vi "Timer Reset.vi"(8 "error in (no error)":errorcluster, 11 "LV Server in":refnum<class "LV Server.lvclass">) -> (0 "error out":errorcluster, 3 "LV Server out":refnum<class "LV Server.lvclass">)   [LabVIEW 2020, in "LV Server.lvclass"]
uses:
  LV Server.lvclass
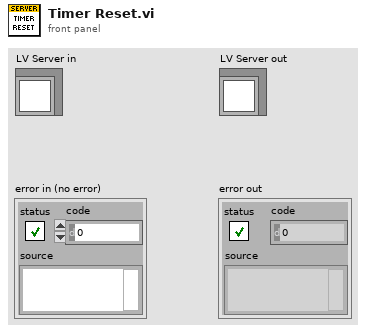
[diagram p1: front panel]
types:
  T1 = typedef "LV Server.lvclass/Timer Data.ctl" = cluster{"Start":dbl, "Accumulated":dbl, "Running":bool}
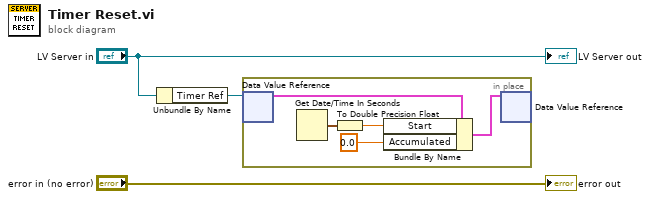
[diagram p0: block diagram]
diagram:
  n1 = Unbundle By Name("LV Server in") -> ("Timer Ref"=w2:refnum<data-value>)
  n2 = in-place {
    n3 = in-place-dvr #1(w2) -> (w7:T1)  [unwired: 1 out]
    n4 = Get Date/Time In Seconds() -> (seconds since 1Jan1904=w6:timestamp)
    n5 = To Double Precision Float(number=w6) -> (double precision float=w5:dbl)
    n6 = Bundle By Name(cluster=w7, "Start"=w5, "Accumulated"=0.0) -> (w8:T1)
    n7 = in-place-dvr #1(w8) -> ()  [unwired: 2 out]
  }
  "error out" <- "error in (no error)"
  "LV Server out" <- "LV Server in"
